vi "1B_AnalyzePulseTrain_wOptions_Sub_Fix1.vi"(0 "Filtered data":waveform(dbl), 1 "Repetitions in the Input Waveform":i32, 5 "Offset":dbl, 7 "Pulse Characteristics":T2) -> (4 "Frequency":dbl, 6 "Avg. CBC Amplitude":dbl, 8 "Stim PW":dbl[](array[numeric]), 9 "Recovery Holdoff":dbl[](array[numeric]), 10 "Waveform Parameters":T1, 11 "Recovery Amplitude":dbl[](array[numeric]), 12 "Stim Amplitude":dbl[](array[numeric]), 13 "Avg. CBC Width":dbl, 14 "Recovery PW":dbl[](array[numeric]), 15 "Interphase Delay":dbl[](array[numeric]))   [LabVIEW 2010]
uses:
  <vilib>/measure/mamon.llb/Trigger Detection for 1 Channel.vi
  <vilib>/measure/NI_MAPro.lvlib
  <vilib>/Analysis/NI_AALBase.lvlib
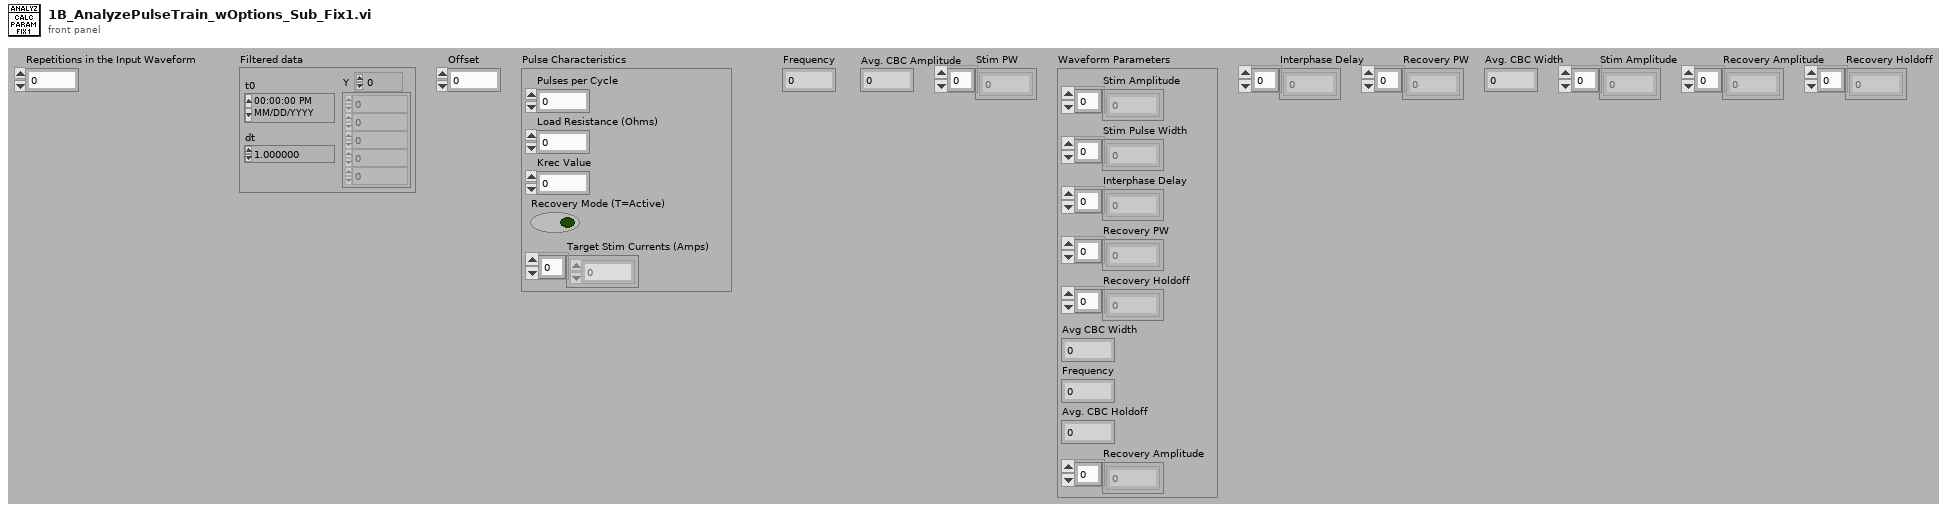
[diagram p1: front panel]
types:
  T1 = cluster{"Stim Amplitude":dbl[], "Stim Pulse Width":dbl[], "Interphase Delay":dbl[], "Recovery PW":dbl[], "Recovery Holdoff":dbl[], "Avg CBC Width":dbl, "Frequency":dbl, "Avg. CBC Holdoff":dbl, "Recovery Amplitude":dbl[]}
  T2 = cluster{"Pulses per Cycle":i32, "Load Resistance (Ohms)":dbl, "Krec Value":i32, "Recovery Mode (T=Active)":bool, "Target Stim Currents (Amps)":dbl[]}
  T3 = cluster{"trigger slope":u16, "Trigger Level":dbl}[]
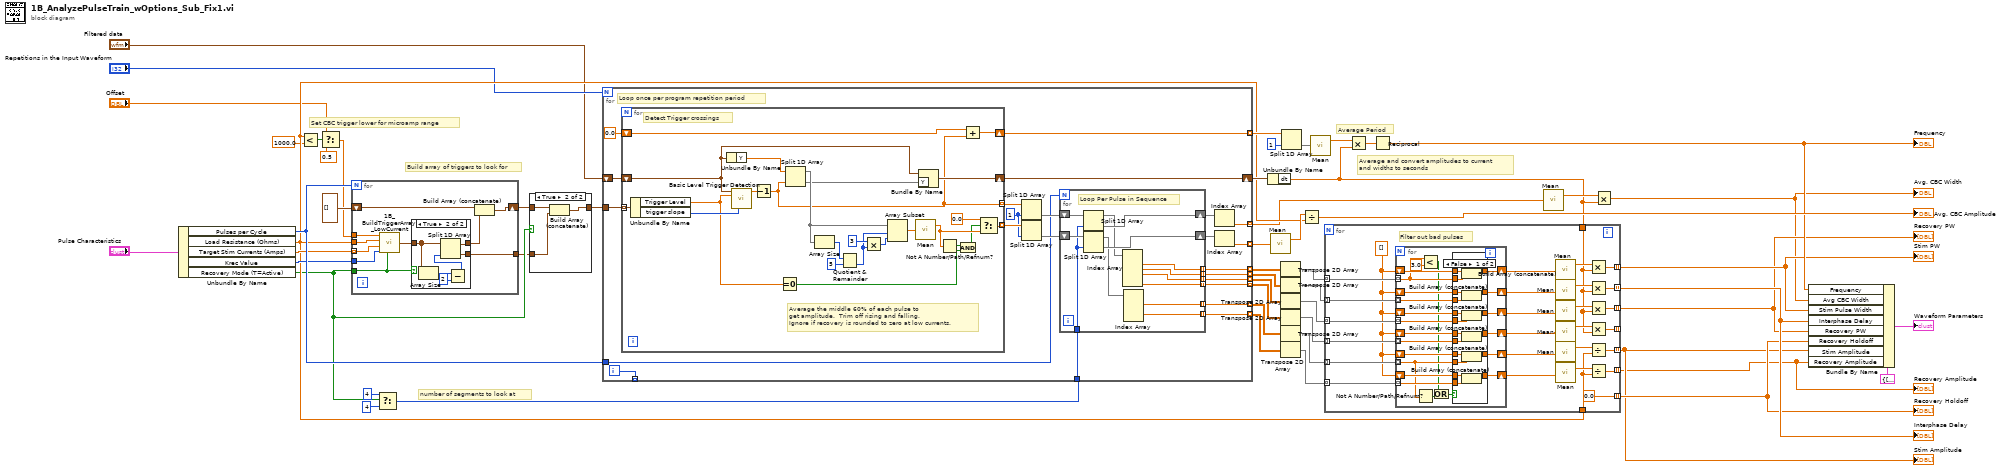
[diagram p0: block diagram]
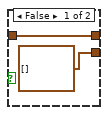
[diagram p4: hidden frame]
diagram:
  # "Set CBC trigger lower for microamp range"
  # "number of segments to look at"
  # "Average Period"
  # "Average and convert amplitudes to current\nand widths to seconds"
  # "Build array of triggers to look for"
  n1 = Unbundle By Name("Pulse Characteristics") -> ("Pulses per Cycle"=w40:i32, "Load Resistance (Ohms)"=w26:dbl, "Target Stim Currents (Amps)"=w27:dbl[], "Krec Value"=w39:i32, "Recovery Mode (T=Active)"=w21:bool)
  n2 = Less?(x=w26, y=1000.0) -> (x < y?=w24:bool)
  n3 = Select(t="Offset", s=w24, f=0.5) -> (s? t:f=w23:dbl)
  n4 = for {
    N: w40 -> [_]
    shift-right: [w64] -> w20
    shift-left: T3 [] -> [w63]
    tunnel: w23 -> [w62]
    tunnel: w21 -> [w58]
    tunnel: w26 -> [w61]
    tunnel: w27 -> [w60] mode=indexing
    tunnel: w39 -> [w59]
    tunnel: [w55] -> w18
    n5 = call "1B_BuildTriggerArray_LowCurrent.vi"("CBC Trigger Level"=w62, "Load Resistance (Ohms)"=w61, "Target Stim Current (Amps)"=w60, "Krec Value"=w59, "Recovery Mode (T=Active)"=w58) -> ("Pulse Triggers"=w57:T3)
    n6 = case shown="True" w58 {
      tunnel: w57 -> [w66 w70]
      tunnel: [w66 w72] -> w56
      tunnel: [T3 [] w71] -> w55
      frame False {
      }
      frame True {
        n7 = Array Size(array=w70) -> (size(s)=w69:i32)
        n8 = Subtract(x=w69, y=2) -> (x-y=w67:i32)
        n9 = Split 1D Array(array=w70, index=w67) -> (first subarray=w72:T3, second subarray=w71:T3)
      }
    }
    n10 = Build Array (concatenate)(w63, w56) -> (w64:T3)
  }
  n11 = Select(t=4, s=w21, f=4 ("index")) -> (s? t:f=w29:i32)
  n12 = case shown="True" w21 {
    tunnel: w20 -> [w73 w76]
    tunnel: [w73 w75] -> w19
    tunnel: w18 -> [_ w74]
    frame False {
    }
    frame True {
      n13 = Build Array (concatenate)(w76, w74) -> (w75:T3)
    }
  }
  n14 = for {
    N: "Repetitions in the Input Waveform" -> [_]
    tunnel: w19 -> [w99]
    shift-right: [w95] -> w38
    shift-left: "Filtered data" -> [w98]
    tunnel: w40 -> [w92]
    tunnel: [w89] -> w4 mode=indexing
    tunnel: [w88] -> w53 mode=indexing
    tunnel: [w87] -> w52 mode=indexing
    tunnel: [w86] -> w51 mode=indexing
    tunnel: [w85] -> w50 mode=indexing
    tunnel: [w84] -> w49 mode=indexing
    tunnel: [w83] -> w48 mode=indexing
    tunnel: [w82] -> w47 mode=indexing
    tunnel: [w79] -> w36 mode=indexing
    tunnel: w29 -> [w78]
    tunnel: [w77] -> _ mode=indexing
    i -> [w77]
    w96 = 1 ("index")
    # "Loop once per program repetition period"
    n15 = for {
      tunnel: w99 -> [w136] mode=indexing
      shift-right: [w125] -> w95
      shift-left: w98 -> [w122]
      tunnel: [w119] -> w97 mode=indexing
      tunnel: [w113] -> w80 mode=indexing
      shift-right: [w128] -> w79
      shift-left: 0.0 -> [w127]
      # "Detect Trigger crossings"
      # "Average the middle 60% of each pulse to\nget amplitude.  Trim off rising and falling.\nIgnore if recovery is rounded to zero at low currents."
      n16 = Unbundle By Name(w136) -> ("Trigger Level"=w120:dbl, "trigger slope"=w126:u16)
      n17 = Unbundle By Name(w122) -> ("Y"=w123:dbl[])
      n18 = call-poly <vilib>:"Basic Level Trigger Detection.vi"("signal in"=w122, "level"=w120, "trigger slope"=w126) -> ("trigger location"=w121:dbl)  [unwired: 10 in, 2 out]
      n19 = Decrement(x=w121) -> (x-1=w113:dbl)
      n20 = Equal To 0?(x=w120) -> (x = 0?=w115:bool)
      n21 = Split 1D Array(array=w123, index=w113) -> (first subarray=w130:dbl[], second subarray=w124:dbl[])
      n22 = Array Size(array=w130) -> (size(s)=w135:i32)
      n23 = Quotient & Remainder(x=w135, y=5) -> (floor(x/y)=w132:i32)  [unwired: 1 out]
      n24 = Multiply(x=3, y=w132) -> (x*y=w131:i32)
      n25 = Array Subset(array=w130, index=w132, length=w131) -> (w129:dbl[])
      n26 = call <vilib>:"Mean.vi"("X"=w129) -> ("mean"=w116:dbl)  [unwired: 1 out]
      n27 = Bundle By Name(cluster=w122, "Y"=w124) -> (w125:waveform(dbl))
      n28 = Not A Number/Path/Refnum?(number/path/refnum=w116) -> (NaN/Path/Refnum?=w117:bool)
      n29 = And(x=w117, y=w115) -> (x .and. y?=w114:bool)
      n30 = Add(x=w127, y=w113) -> (x+y=w128:dbl)
      n31 = Select(t=0.0, s=w114, f=w116) -> (s? t:f=w119:dbl)
    }
    n32 = Split 1D Array(array=w80, index=w96) -> (second subarray=w94:dbl[])  [unwired: 1 out]
    n33 = Split 1D Array(array=w97, index=w96) -> (second subarray=w93:dbl[])  [unwired: 1 out]
    n34 = for {
      N: w92 -> [_]
      shift-right: [w110] -> w91
      shift-left: w94 -> [w112]
      shift-right: [w109] -> w90
      shift-left: w93 -> [w111]
      tunnel: [w106] -> w87 mode=indexing
      tunnel: [w105] -> w86 mode=indexing
      tunnel: [w104] -> w85 mode=indexing
      tunnel: [w100] -> w84 mode=indexing
      tunnel: [w103] -> w83 mode=indexing
      tunnel: [w102] -> w82 mode=indexing
      tunnel: w78 -> [w101]
      # "Loop Per Pulse in Sequence"
      n35 = Split 1D Array(array=w112, index=w101) -> (first subarray=w108:dbl[], second subarray=w110:dbl[])
      n36 = Split 1D Array(array=w111, index=w101) -> (first subarray=w107:dbl[], second subarray=w109:dbl[])
      n37 = Index Array(array=w108) -> (element #1=w106:dbl, element #2=w105:dbl, element #3=w104:dbl, element #5=w100:dbl)  [unwired: 5 in, 1 out]
      n38 = Index Array(array=w107) -> (element #1=w103:dbl, element #3=w102:dbl)  [unwired: 4 in, 2 out]
    }
    n39 = Index Array(array=w91) -> (element=w89:dbl)  [unwired: 1 in]
    n40 = Index Array(array=w90) -> (element=w88:dbl)  [unwired: 1 in]
  }
  n41 = Unbundle By Name(w38) -> ("dt"=w2:dbl)
  n42 = call <vilib>:"Mean.vi"("X"=w53) -> ("mean"=w37:dbl)  [unwired: 1 out]
  n43 = Transpose 2D Array(2D array=w52) -> (transposed array=w46:dbl[][])
  n44 = Transpose 2D Array(2D array=w51) -> (transposed array=w45:dbl[][])
  n45 = Transpose 2D Array(2D array=w50) -> (transposed array=w44:dbl[][])
  n46 = Transpose 2D Array(2D array=w49) -> (transposed array=w43:dbl[][])
  n47 = Transpose 2D Array(2D array=w48) -> (transposed array=w42:dbl[][])
  n48 = Transpose 2D Array(2D array=w47) -> (transposed array=w41:dbl[][])
  n49 = Split 1D Array(array=w36, index=1) -> (second subarray=w35:dbl[])  [unwired: 1 out]
  n50 = Divide(x=w37, y=w26) -> (x/y=→"Avg. CBC Amplitude":dbl)
  n51 = call <vilib>:"Mean.vi"("X"=w35) -> ("mean"=w34:dbl)  [unwired: 1 out]
  n52 = for {
    tunnel: w46 -> [w144] mode=indexing
    tunnel: w45 -> [w149] mode=indexing
    tunnel: w44 -> [w148] mode=indexing
    tunnel: w43 -> [w147] mode=indexing
    tunnel: w42 -> [w146] mode=indexing
    tunnel: w41 -> [w145] mode=indexing
    tunnel: [w164] -> w10 mode=indexing
    tunnel: [w163] -> w9 mode=indexing
    tunnel: [w162] -> w8 mode=indexing
    tunnel: [w161] -> _ mode=indexing
    tunnel: [w160] -> w6 mode=indexing
    tunnel: [w159] -> w5 mode=indexing
    tunnel: w2 -> [w152]
    tunnel: w26 -> [w151]
    tunnel: [0.0 ("Load Resistance (Ohms)")] -> w7 mode=indexing
    w143 = dbl[] []
    # "Filter out bad pulses"
    n53 = for {
      tunnel: w144 -> [w167] mode=indexing
      tunnel: w149 -> [w174] mode=indexing
      tunnel: w148 -> [w173] mode=indexing
      tunnel: w147 -> [w172] mode=indexing
      tunnel: w146 -> [w170] mode=indexing
      tunnel: w145 -> [w171] mode=indexing
      shift-right: [w185] -> w142
      shift-left: w143 -> [w186]
      shift-right: [w183] -> w141
      shift-left: w143 -> [w184]
      shift-right: [w181] -> w140
      shift-left: w143 -> [w182]
      shift-right: [w179] -> w139
      shift-left: w143 -> [w180]
      shift-right: [w177] -> w138
      shift-left: w143 -> [w178]
      shift-right: [w175] -> w137
      shift-left: w143 -> [w176]
      n54 = Not A Number/Path/Refnum?(number/path/refnum=w170) -> (NaN/Path/Refnum?=w168:bool)
      n55 = Less?(x=w167, y=3.0) -> (x < y?=w165:bool)
      n56 = Or(x=w165, y=w168) -> (x .or. y?=w169:bool)
      n57 = case shown="False" w169 {
        tunnel: w186 -> [w202 w210]
        tunnel: [w203 w210] -> w185
        tunnel: w184 -> [w191 w209]
        tunnel: [w196 w209] -> w183
        tunnel: w182 -> [w190 w208]
        tunnel: [w195 w208] -> w181
        tunnel: w180 -> [w189 w207]
        tunnel: [w194 w207] -> w179
        tunnel: w178 -> [w188 w206]
        tunnel: [w193 w206] -> w177
        tunnel: w176 -> [w187 w205]
        tunnel: [w192 w205] -> w175
        tunnel: w167 -> [w204 _]
        tunnel: w174 -> [w201 _]
        tunnel: w173 -> [w200 _]
        tunnel: w172 -> [w199 _]
        tunnel: w170 -> [w198 _]
        tunnel: w171 -> [w197 _]
        frame False {
          n58 = Build Array (concatenate)(w191, w201) -> (w196:dbl[])
          n59 = Build Array (concatenate)(w190, w200) -> (w195:dbl[])
          n60 = Build Array (concatenate)(w189, w199) -> (w194:dbl[])
          n61 = Build Array (concatenate)(w188, w198) -> (w193:dbl[])
          n62 = Build Array (concatenate)(w202, w204) -> (w203:dbl[])
          n63 = Build Array (concatenate)(w187, w197) -> (w192:dbl[])
        }
        frame True {
        }
      }
    }
    n64 = call <vilib>:"Mean.vi"("X"=w142) -> ("mean"=w157:dbl)  [unwired: 1 out]
    n65 = call <vilib>:"Mean.vi"("X"=w141) -> ("mean"=w156:dbl)  [unwired: 1 out]
    n66 = call <vilib>:"Mean.vi"("X"=w140) -> ("mean"=w155:dbl)  [unwired: 1 out]
    n67 = call <vilib>:"Mean.vi"("X"=w139) -> ("mean"=w154:dbl)  [unwired: 1 out]
    n68 = call <vilib>:"Mean.vi"("X"=w138) -> ("mean"=w153:dbl)  [unwired: 1 out]
    n69 = call <vilib>:"Mean.vi"("X"=w137) -> ("mean"=w158:dbl)  [unwired: 1 out]
    n70 = Multiply(x=w157, y=w152) -> (x*y=w164:dbl)
    n71 = Multiply(x=w156, y=w152) -> (x*y=w163:dbl)
    n72 = Multiply(x=w155, y=w152) -> (x*y=w162:dbl)
    n73 = Multiply(x=w154, y=w152) -> (x*y=w161:dbl)
    n74 = Divide(x=w153, y=w151) -> (x/y=w160:dbl)
    n75 = Divide(x=w158, y=w151) -> (x/y=w159:dbl)
  }
  "Stim PW" <- w10
  "Interphase Delay" <- w9
  "Recovery PW" <- w8
  "Recovery Holdoff" <- w7
  "Stim Amplitude" <- w6
  "Recovery Amplitude" <- w5
  n76 = Multiply(x=w34, y=w2) -> (x*y=w33:dbl)
  n77 = Reciprocal(x=w33) -> (1/x=w11:dbl)
  "Frequency" <- w11
  n78 = call <vilib>:"Mean.vi"("X"=w4) -> ("mean"=w3:dbl)  [unwired: 1 out]
  n79 = Multiply(x=w3, y=w2) -> (x*y=w1:dbl)
  "Avg. CBC Width" <- w1
  n80 = Bundle By Name(cluster=T1 {"Stim Amplitude"=[], "Stim Pulse Width"=[], "Interphase Delay"=[], "Recovery PW"=[], "Recovery Holdoff"=[], "Avg CBC Width"=0.0, "Frequency"=0.0, "Avg. CBC Holdoff"=0.0, "Recovery Amplitude"=[]} ("Pulse Train Parameters"), "Frequency"=w11, "Avg CBC Width"=w1, "Stim Pulse Width"=w10, "Interphase Delay"=w9, "Recovery PW"=w8, "Recovery Holdoff"=w7, "Stim Amplitude"=w6, "Recovery Amplitude"=w5) -> (→"Waveform Parameters":T1)
